vi "UTIL Probe.vi"(8 "error in (no error)":errorcluster, 11 "niDTS Comm String in":refnum<class "niDTS Comm String.lvclass">) -> (0 "error out":errorcluster, 3 "niDTS Comm String out":refnum<class "niDTS Comm String.lvclass">)   [LabVIEW 2015, in "niDTS CommLib.lvlib" / "niDTS Comm String.lvclass"]
uses:
  niDTS Comm String.lvclass
  Includes/niDTS Comm INC CLI Login.ctl
  niDTS Comm String.lvclass/niDTS Comm String.ctl
  niDTS CommLib.lvlib
panel:
  out "waitForAckEnabled":bool=TRUE
  out "loggingEnabled":bool=TRUE
  out "readEnabled":bool=TRUE
  out "portName":string
  out "lastRead":string
  out "cmdPrefix":string
  out "CLI Login":T1
  out "ACK":string
  out "ACKTimeout":i32
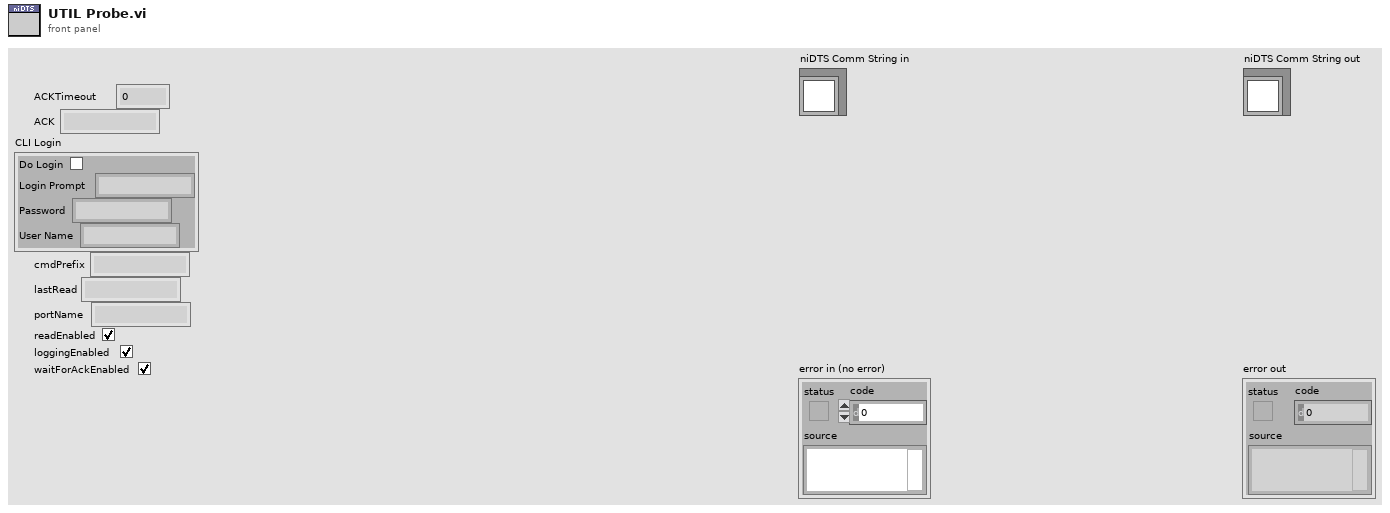
[diagram p1: front panel]
types:
  T1 = typedef "niDTS CommLib.lvlib/niDTS Comm INC CLI Login.ctl" = cluster{"Do Login":bool, "Login Prompt":string, "Password":string, "User Name":string}
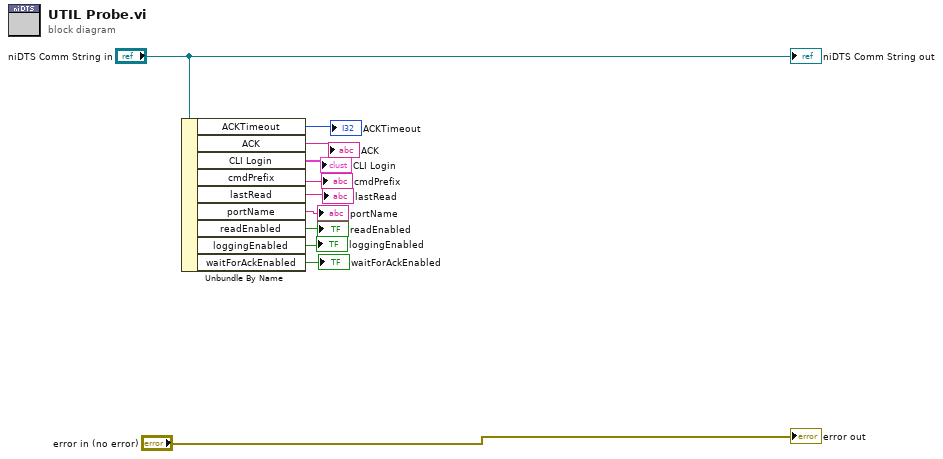
[diagram p0: block diagram]
diagram:
  n1 = Unbundle By Name("niDTS Comm String in") -> ("ACKTimeout"=→"ACKTimeout":i32, "ACK"=→"ACK":string, "CLI Login"=→"CLI Login":T1, "cmdPrefix"=→"cmdPrefix":string, "lastRead"=→"lastRead":string, "portName"=→"portName":string, "readEnabled"=→"readEnabled":bool, "loggingEnabled"=→"loggingEnabled":bool, "waitForAckEnabled"=→"waitForAckEnabled":bool)
  "error out" <- "error in (no error)"
  "niDTS Comm String out" <- "niDTS Comm String in"
